vi "exportToExcel.vi"(11 "Export Data":string[][](array[string])) -> ()   [LabVIEW 2017]
doc: "This example uses the \"Register ActiveX Event Callback\" with a Microsoft Excel ActiveX control. \nIt demonstrates how to register an event and extract event data."
uses:
  <vilib>/Utility/file.llb/Write To Spreadsheet File (string).vi
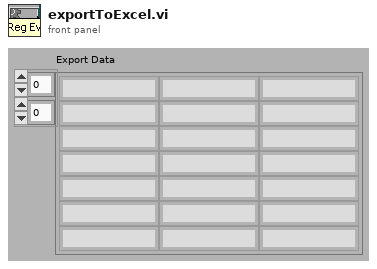
[diagram p1: front panel]
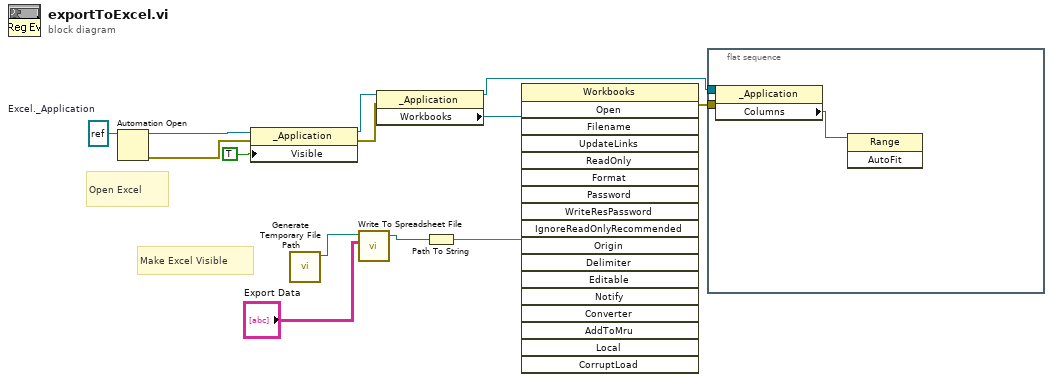
[diagram p0: block diagram]
diagram:
  w13 = refnum<k7> refnum  # Excel._Application
  # "Make Excel Visible"
  # "Open Excel"
  n1 = Automation Open(Automation Refnum=w13) -> (Automation Refnum=w11:refnum<k7>, error out=w8:errorcluster)  [unwired: 3 in]
  n2 = property on="Property Node" class="_Application"(reference=w11, error in=w8, "Visible"=TRUE) -> (reference out=w10:refnum<k7>, error out=w9:errorcluster)
  n3 = call <vilib>:"Generate Temporary File Path.vi"() -> ("Unique Temporary File Path"=w7:path)  [unwired: 10 in, 1 out]
  n4 = call-poly <vilib>:"Write To Spreadsheet File.vi"("2D data"="Export Data", "file path (dialog if empty)"=w7) -> ("new file path (Not A Path if cancelled)"=w4:path)  [unwired: 6 in]
  n5 = property class="_Application"(reference=w10, error in=w9) -> (reference out=w2:refnum<k7>, "Workbooks"=w5:refnum<k7>)  [unwired: 1 out]
  n6 = Path To String(path=w4) -> (string=w3:string)
  n7 = invoke class="Workbooks" method="Open"(reference=w5, "Filename"=w3) -> (error out=w1:errorcluster)  [unwired: 16 in, 17 out]
  n8 = flat-sequence {
    tunnel: w2 -> [w15]
    tunnel: w1 -> [_]
    frame #0 {
      n9 = property class="_Application"(reference=w15) -> ("Columns"=w14:refnum<k7>)  [unwired: 1 in, 2 out]
      n10 = invoke class="Range" method="AutoFit"(reference=w14) -> ()  [unwired: 2 in, 3 out]
    }
  }
